vi "HEAVE UDP TRIAL.vi"() -> ()   [LabVIEW 2025]
panel:
  out "connection ID out":refnum<k16>
  in  "Checkbox":bool
  in  "Fine Tune Zone":dbl=10.0
  out "Pulse delta":dbl
  in  "seconds to wait 3":dbl=1.0 format="%#_6p"
  in  "Max_pos_limit":dbl=50000000.0
  in  "Min_pos_limit":dbl
  in  "i_limit":dbl=10.0
  in  "Max Step Linit":dbl=10.0
  in  "Init Step":dbl=10.0
  in  "pct_scale":dbl=100.0
  in  "Deadband":dbl=0.1
  in  "Kd":dbl
  in  "Ki":dbl
  in  "Kp":dbl=1.0
  out "Current Position":dbl
  in  "Set Load":dbl
  in  "Current Load":dbl
  out "Node Id":u8
  in  "PID SPEED":sgl=80000.0
  in  "PID":bool
  in  "seconds to wait 2":dbl=0.2 format="%#_6p"
  out "Pulse Output":dbl
  out "Trigger":dbl
  in  "Low Command":dbl
  in  "High Command":dbl=10000.0
  in  "Time Low":dbl=1.5
  in  "Time High":dbl=1.5
  in  "dt":dbl=0.01
  out "fwMinor":u8
  out "fwMajor":u8
  out "faultCode":u16
  out "SURGE POSE":sgl format="%#.6f"
  out "HEAVE POSE":sgl format="%#.6f"
  out "Homed":u8
  out "State":u8
  out "Ack ID":u16
  in  "Write":bool
  in  "Read":bool
  in  "seconds to wait":dbl=0.001 format="%#_6p"
  in  "SPEED":sgl=10000.0
  in  "Distance":sgl=10000.0
  in  "Mode Command":u8=2
  out "Sequence ID":u16=7
  out "string 2":string
  in  "Stop Button":bool
  in  "Server Name":string="192.168.1.10"
  out "data out 2":string
  # "0100 0100 0000 0000 0000 0000 0000 00"
  # "0100 0100 0000 0000 0000 0000 0000 0000"
  # "0500 0501 40C2 0C48 0000 0000 0000 0100"
  # "0300 0301 00CB E547 0000 0000 0000 0100"
  # "Home"
  # "0100 0100 0000 0000 0000 00"
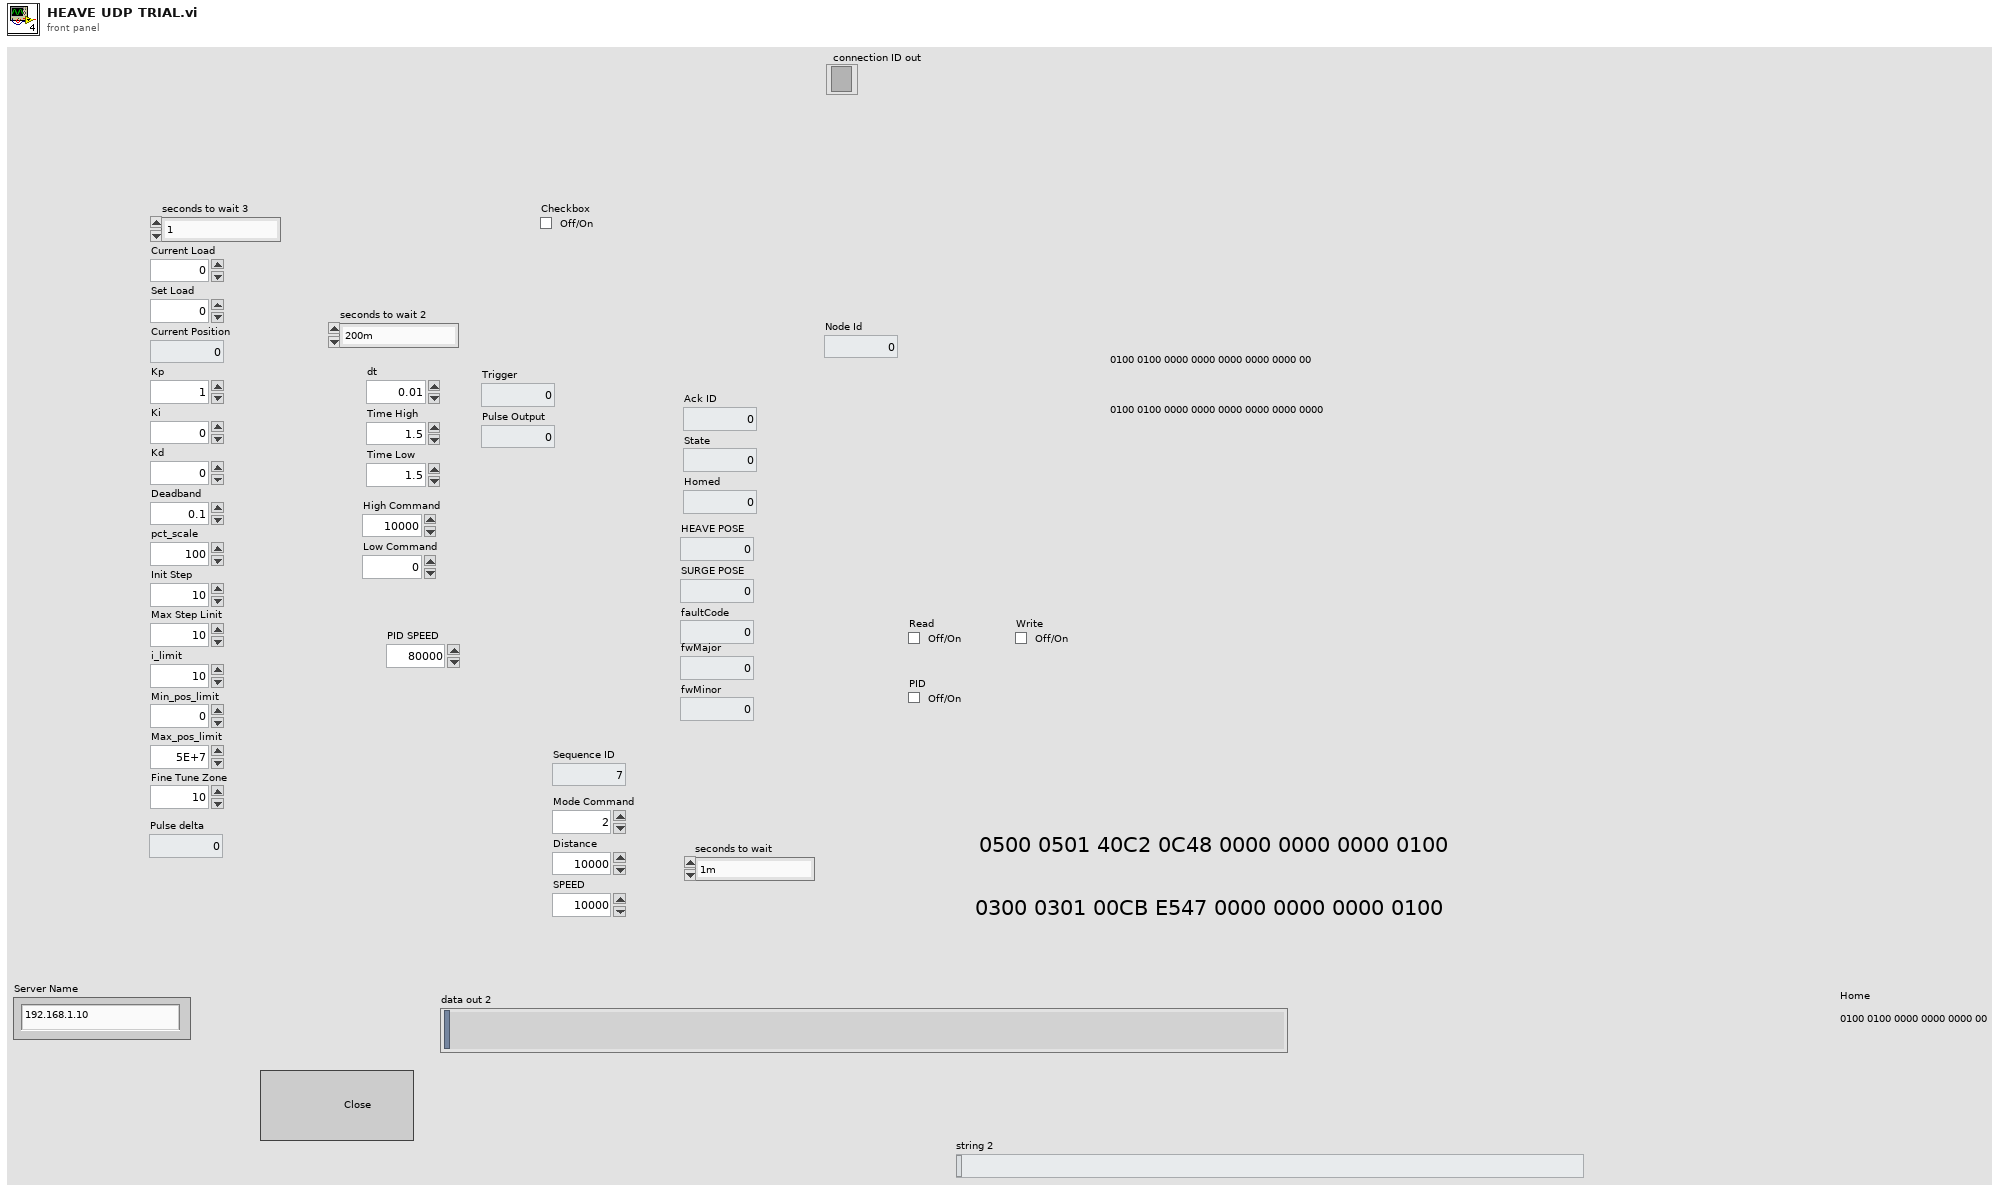
[diagram p1: front panel]
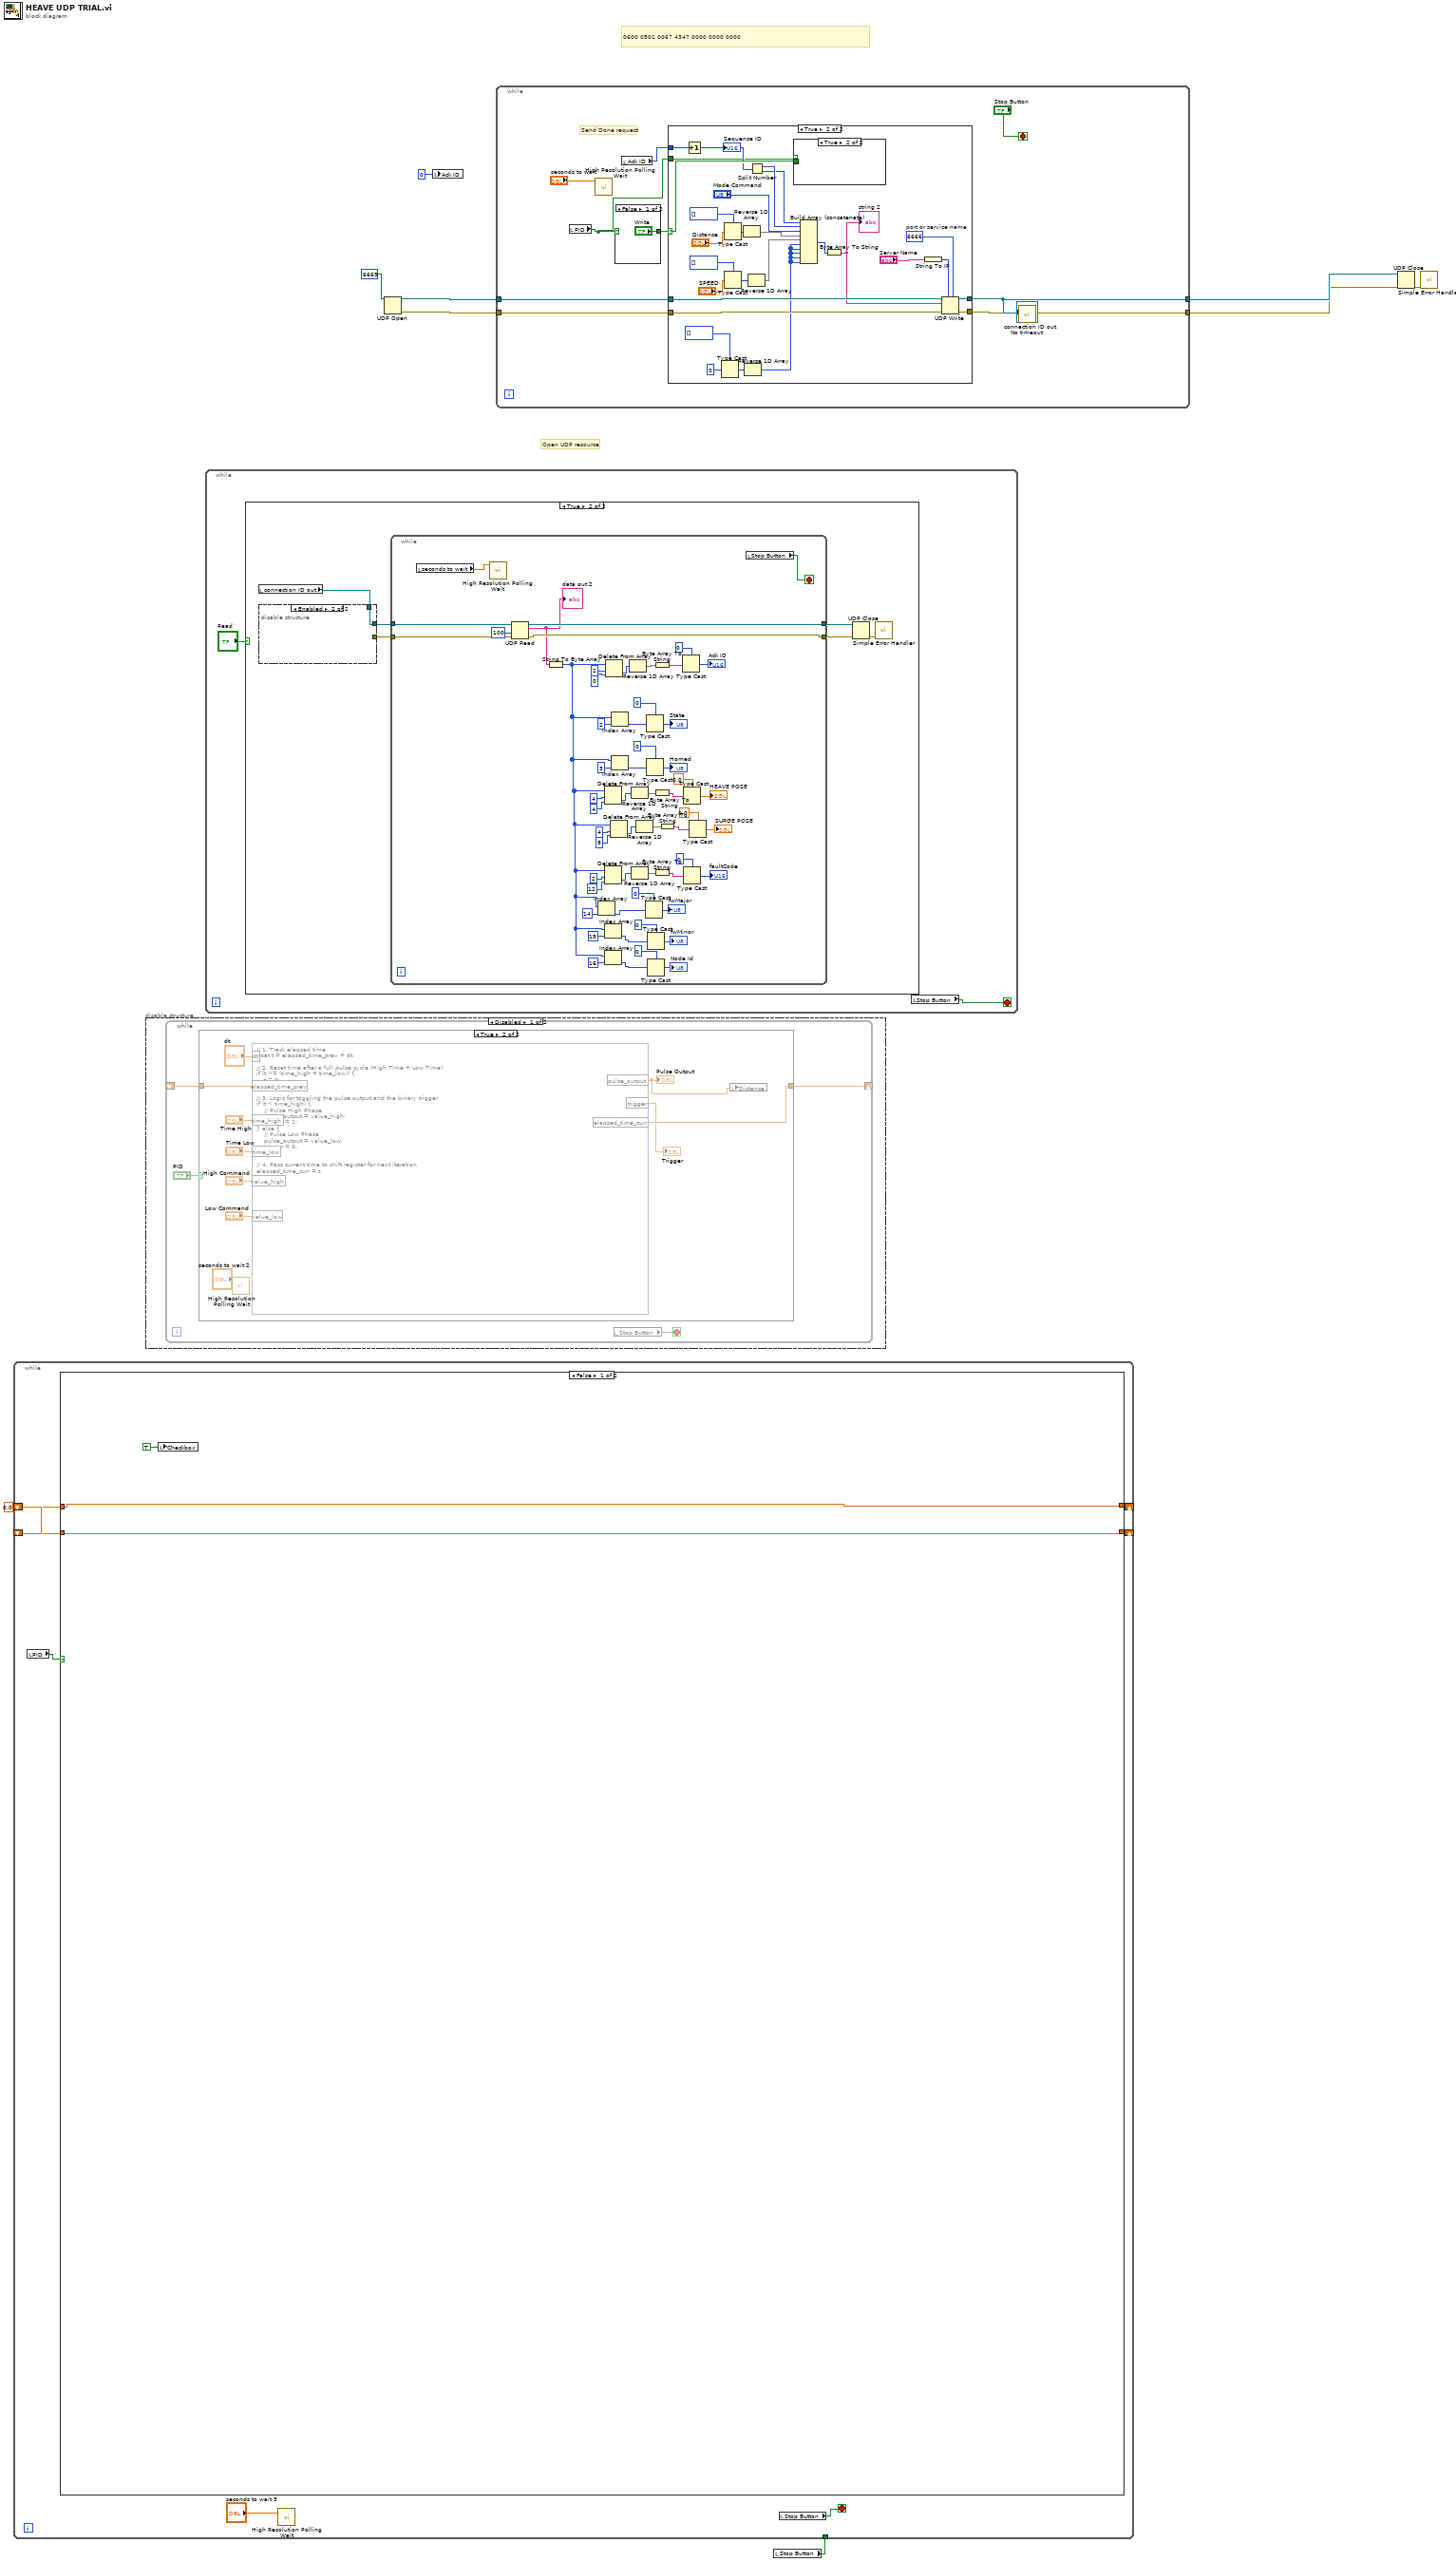
[diagram p0: block diagram]
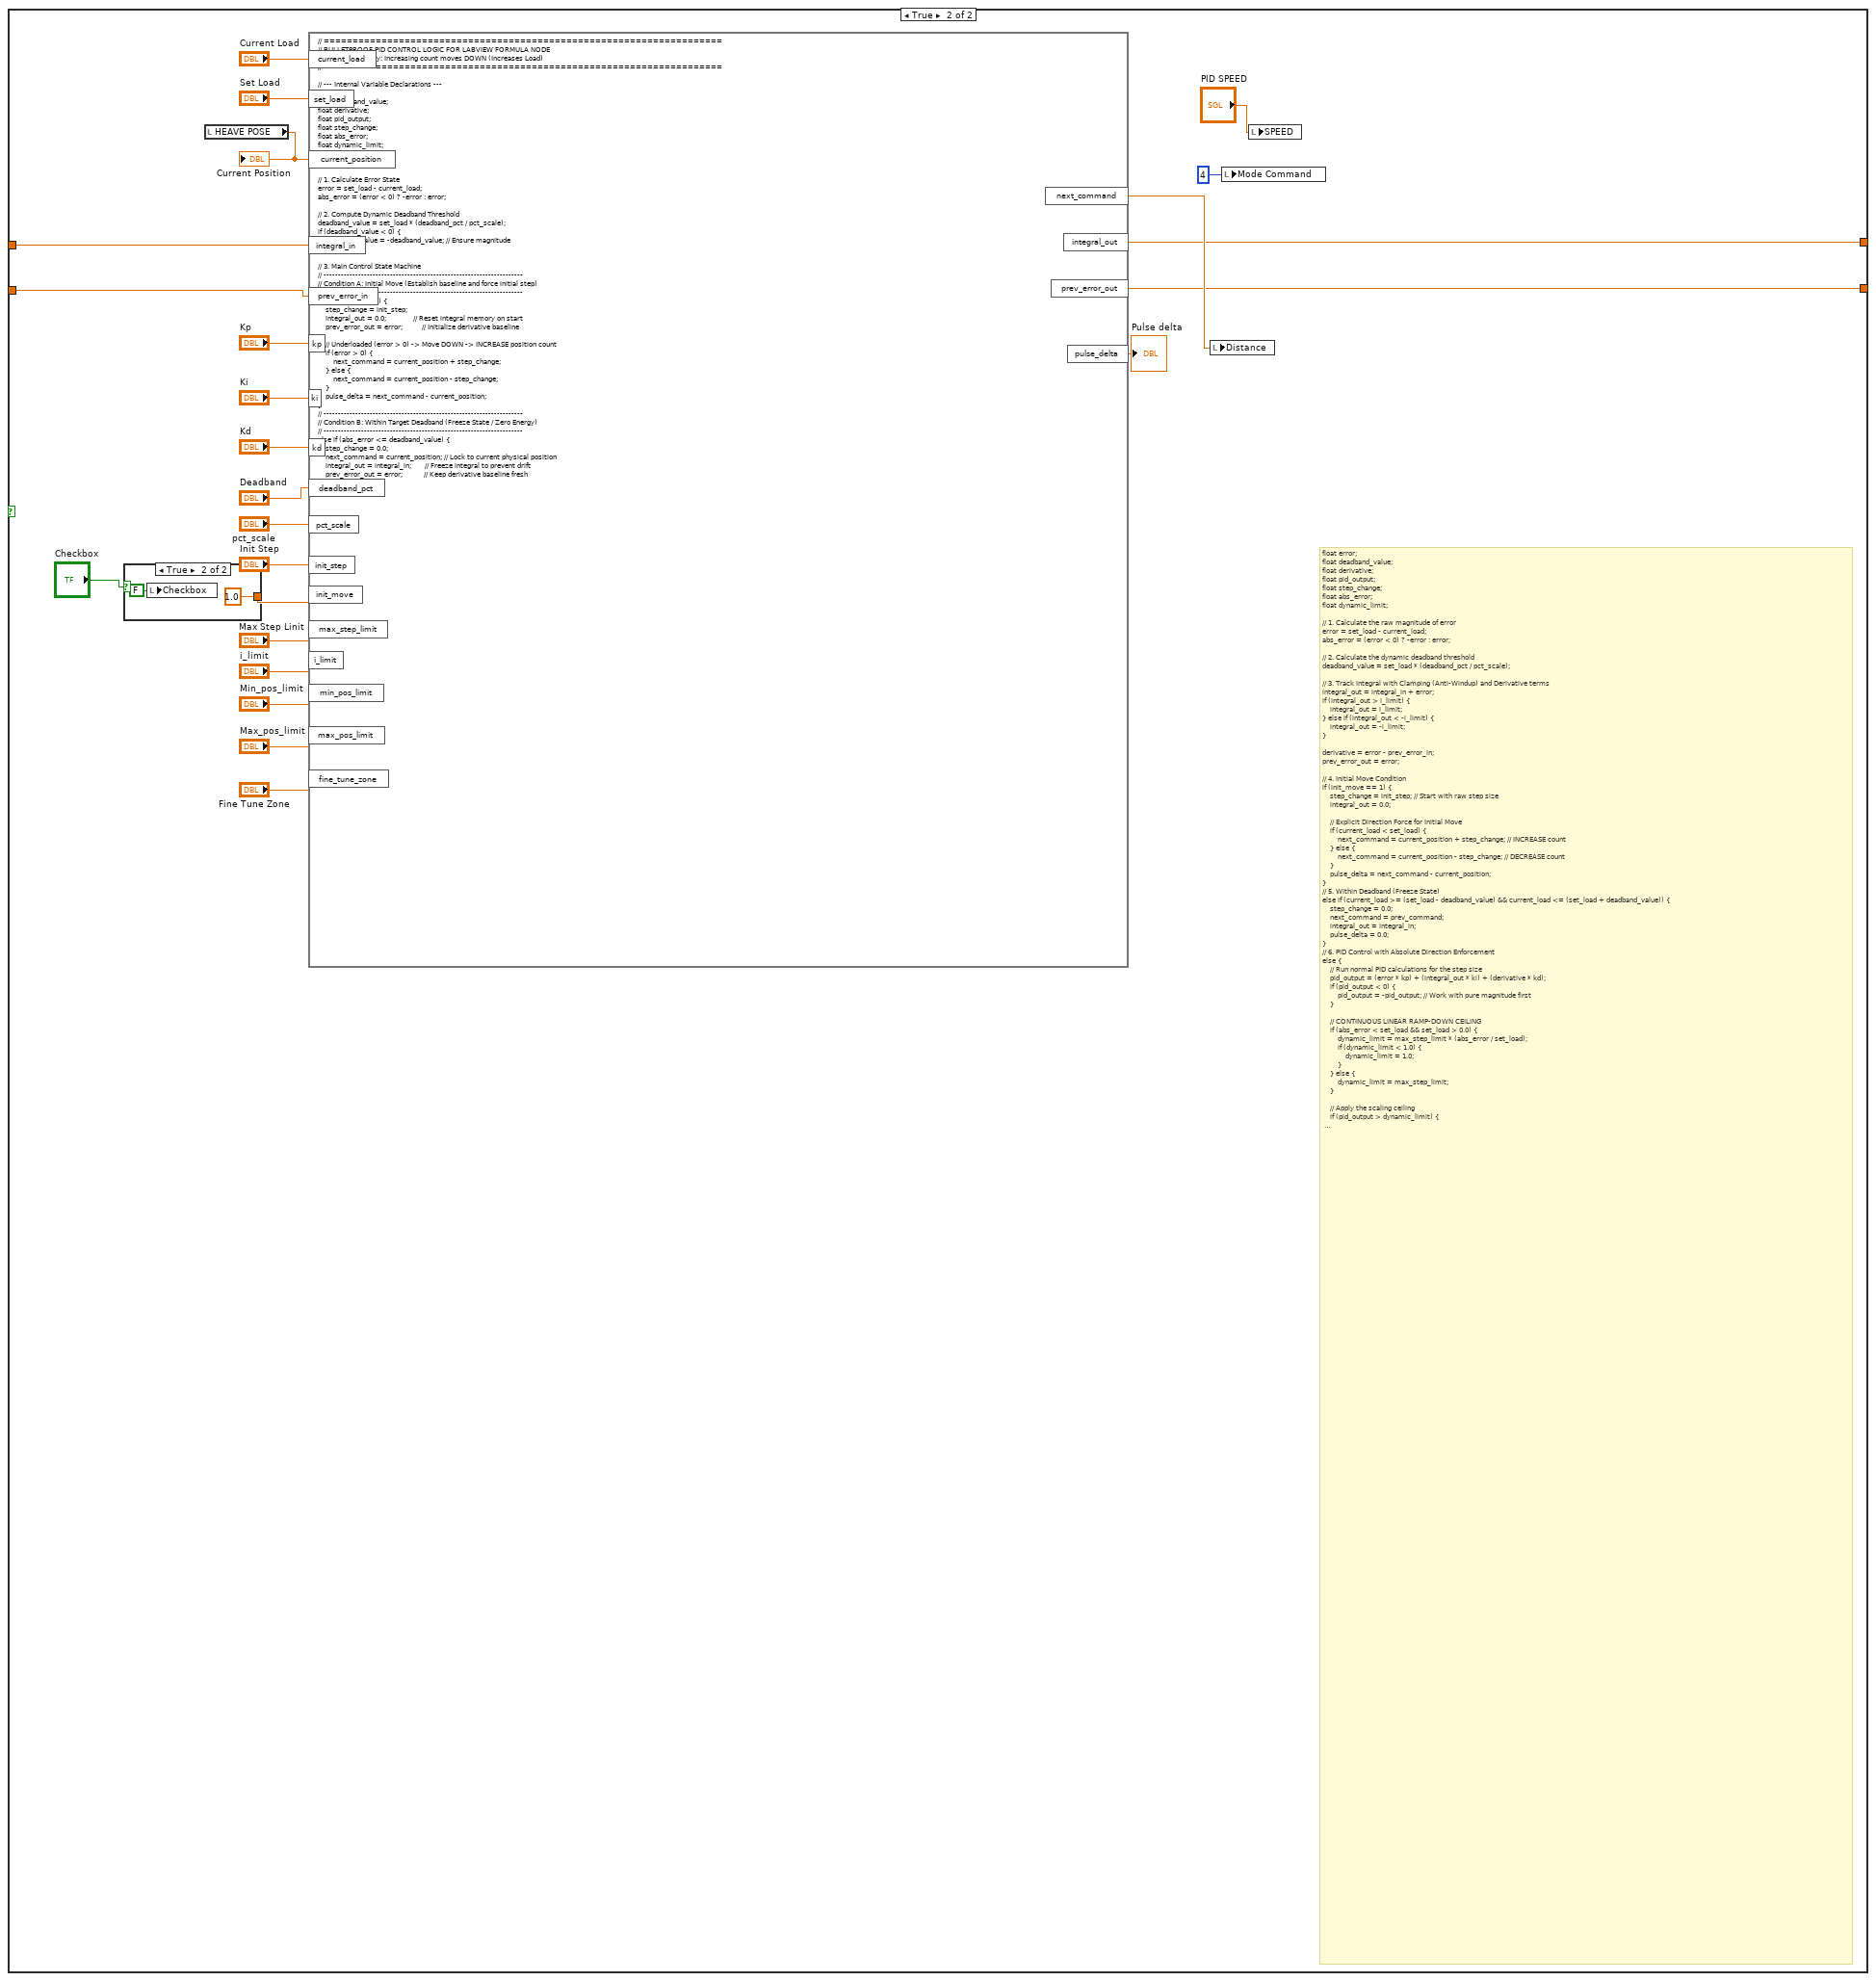
[diagram p2: hidden frame]
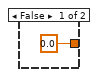
[diagram p3: hidden frame]
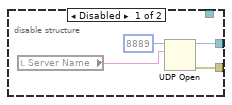
[diagram p7: hidden frame]
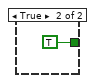
[diagram p8: hidden frame]
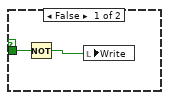
[diagram p10: hidden frame]
diagram:
  w1 = 0.0 ("integral_out")
  # "0600 0501 0067 4347 0000 0000 0000"
  # "Open UDP resource"
  n1 = disable-structure shown="Disabled" {
    frame Disabled {
      n2 = while {
        shift-right: [w11] -> _
        shift-left: _ -> [w12]
        stop <- w13 stop-if-true
        n3 = case shown="True" "PID" {
          tunnel: w12 -> [w14 w23]
          tunnel: [w14 w22] -> w11
          frame False {
          }
          frame True {
            n4 = call <vilib>:"High Resolution Polling Wait.vi"("seconds to wait"="seconds to wait 2") -> ()  [unwired: 10 in, 1 out]
            n5 = formula code="// 1. Track elapsed time\nfloat t = elapsed_time_prev + dt;\n\n// 2. Reset time after a full pulse cycle (High Time + Low Time)\nif (t >= (time_high + time_low)) {\n    t = 0;\n}\n\n// 3. Logic for toggling the pulse output and the binary trigger\nif (t < time_high) {\n    // Pulse High Phase\n    pulse_output = value_high;\n    trigger = 1; \n} else {\n    // Pulse Low Phase\n    pulse_output = value_low;\n    trigger = 0;\n}\n\n// 4. Pass current time to shift register for next iteration\nelapsed_time_curr = t;"("dt"="dt", "elapsed_time_prev"=w23, "time_high"="Time High", "time_low"="Time Low", "value_high"="High Command", "value_low"="Low Command") -> ("pulse_output"=w15:dbl, "trigger"=→"Trigger":dbl, "elapsed_time_curr"=w22:dbl)
            "Pulse Output" <- w15
            n6 = local write "Distance"(w15) -> ()
          }
        }
        n7 = local read "Stop Button"() -> (w13:bool)
      }
    }
    frame Enabled {
    }
  }
  n8 = while {
    stop <- w25 stop-if-true
    n9 = case shown="True" "Read" {
      frame False {
      }
      frame True {
        n10 = local read "connection ID out"() -> (w27:refnum<k16>)
        n11 = disable-structure shown="Enabled" {
          disable-tunnel: [w35 _] -> w32
          disable-tunnel: [w34 w37] -> w31
          disable-tunnel: w27 -> [_ w37]
          frame Disabled {
            n12 = local read "Server Name"() -> (w33:string)
            n13 = UDP Open(10:w33, 11:u16 8889 ("port")) -> (port=w34:refnum<k16>, 0:w35:errorcluster)  [unwired: 3 in, 1 out]
          }
          frame Enabled {
          }
        }
        n14 = while {
          tunnel: w32 -> [w94]
          tunnel: w31 -> [w93]
          tunnel: [w92] -> w29
          tunnel: [w90] -> w28
          stop <- w91 stop-if-true
          n15 = local read "seconds to wait"() -> (w88:dbl)
          n16 = call <vilib>:"High Resolution Polling Wait.vi"("seconds to wait"=w88) -> ()  [unwired: 10 in, 1 out]
          n17 = UDP Read(connection ID=w93, timeout ms (25000)=100, 8:w94) -> (data out=w47:string, error out=w92:errorcluster, 3:w90:refnum<k16>)  [unwired: 1 in, 2 out]
          "data out 2" <- w47
          n18 = String To Byte Array(string=w47) -> (unsigned byte array=w38:u8[])
          n19 = Index Array(array=w38, index=14) -> (element=w51:u8)
          n20 = Delete From Array(array=w38, length=4, index=4) -> (deleted portion=w43:u8[])  [unwired: 1 out]
          n21 = Delete From Array(array=w38, length=2, index=12) -> (deleted portion=w44:u8[])  [unwired: 1 out]
          n22 = Index Array(array=w38, index=15) -> (element=w48:u8)
          n23 = Index Array(array=w38, index=16) -> (element=w42:u8)
          n24 = Delete From Array(array=w38, length=2, index=0) -> (deleted portion=w45:u8[])  [unwired: 1 out]
          n25 = Delete From Array(array=w38, length=4, index=8) -> (deleted portion=w46:u8[])  [unwired: 1 out]
          n26 = Index Array(array=w38, index=2) -> (element=w79:u8)
          n27 = Index Array(array=w38, index=3) -> (element=w76:u8)
          n28 = Reverse 1D Array(array=w45) -> (reversed array=w85:u8[])
          n29 = Reverse 1D Array(array=w43) -> (reversed array=w71:u8[])
          n30 = Reverse 1D Array(array=w44) -> (reversed array=w58:u8[])
          n31 = Reverse 1D Array(array=w46) -> (reversed array=w66:u8[])
          n32 = Type Cast(type=u8 0, x=w51) -> (*(type *) &x=→"fwMajor":u8)
          n33 = Type Cast(type=u8 0, x=w79) -> (*(type *) &x=→"State":u8)
          n34 = Type Cast(type=u8 0, x=w76) -> (*(type *) &x=→"Homed":u8)
          n35 = Type Cast(type=u8 0, x=w48) -> (*(type *) &x=→"fwMinor":u8)
          n36 = Type Cast(type=u8 0, x=w42) -> (*(type *) &x=→"Node Id":u8)
          n37 = Byte Array To String(unsigned byte array=w71) -> (string=w69:string)
          n38 = Byte Array To String(unsigned byte array=w58) -> (string=w57:string)
          n39 = Byte Array To String(unsigned byte array=w85) -> (string=w83:string)
          n40 = Byte Array To String(unsigned byte array=w66) -> (string=w67:string)
          n41 = Type Cast(type=u16 0, x=w83) -> (*(type *) &x=→"Ack ID":u16)
          n42 = Type Cast(type=sgl 0.0, x=w69) -> (*(type *) &x=→"HEAVE POSE":sgl)
          n43 = Type Cast(type=u16 0, x=w57) -> (*(type *) &x=→"faultCode":u16)
          n44 = Type Cast(type=sgl 0.0, x=w67) -> (*(type *) &x=→"SURGE POSE":sgl)
          n45 = local read "Stop Button"() -> (w91:bool)
        }
        n46 = UDP Close(connection ID=w28, 8:w29) -> (error out=w30:errorcluster)  [unwired: 1 out]
        n47 = call <vilib>:"Simple Error Handler.vi"("error in (no error)"=w30) -> ()  [unwired: 4 in, 5 out]
      }
    }
    n48 = local read "Stop Button"() -> (w25:bool)
  }
  n49 = UDP Open(11:u16 6669 ("port")) -> (port=w9:refnum<k16>, 0:w8:errorcluster)  [unwired: 4 in, 1 out]
  n50 = local write "Ack ID"(u16 0 ("Ack ID")) -> ()
  n51 = while {
    tunnel: w9 -> [w104]
    tunnel: w8 -> [w103]
    tunnel: [w101] -> w6
    tunnel: [w102] -> w5
    stop <- "Stop Button" stop-if-true
    # "Send Done request"
    n52 = local read "PID"() -> (w95:bool)
    n53 = call <vilib>:"High Resolution Polling Wait.vi"("seconds to wait"="seconds to wait") -> ()  [unwired: 10 in, 1 out]
    n54 = case shown="False" w95 {
      tunnel: ["Write" TRUE ("Write")] -> w97
      frame False {
      }
      frame True {
      }
    }
    n55 = local read "Ack ID"() -> (w96:u16)
    n56 = case shown="True" w97 {
      selector: w97 -> [_ w116]
      tunnel: w104 -> [w107 w136]
      tunnel: w103 -> [w108 w135]
      tunnel: [w107 w132] -> w101
      tunnel: [w108 w131] -> w100
      tunnel: w96 -> [_ w115]
      tunnel: w95 -> [_ w113]
      frame False {
      }
      frame True {
        w130 = u16 6666  # port or service name
        n57 = Increment(x=w115) -> (x+1=w114:u16)
        "Sequence ID" <- w114
        n58 = Type Cast(type=u8[] [], x=u8 0) -> (*(type *) &x=w112:u8[])
        n59 = Type Cast(type=u8[] [], x="Distance") -> (*(type *) &x=w123:u8[])
        n60 = Type Cast(type=u8[] [], x="SPEED") -> (*(type *) &x=w124:u8[])
        n61 = Reverse 1D Array(array=w123) -> (reversed array=w128:u8[])
        n62 = Reverse 1D Array(array=w112) -> (reversed array=w109:u8[])
        n63 = Reverse 1D Array(array=w124) -> (reversed array=w129:u8[])
        n64 = Split Number(x=w114) -> (hi(x)=w127:u8, lo(x)=w126:u8)
        n65 = case shown="True" w113 {
          tunnel: w116 -> [w138 _]
          frame False {
            n66 = Not(x=w138) -> (.not. x?=w137:bool)
            n67 = local write "Write"(w137) -> ()
          }
          frame True {
          }
        }
        n68 = Build Array (concatenate)(w126, w127, "Mode Command", w128, w129, w109, w109, w109, w109, w109) -> (w125:u8[])
        n69 = Byte Array To String(unsigned byte array=w125) -> (string=w119:string)
        "string 2" <- w119
        n70 = String To IP(1:"Server Name") -> (0:w133:u32)
        n71 = UDP Write(address=w133, port or service name=w130, connection ID=w136, data in=w119, 8:w135) -> (error out=w131:errorcluster, 3:w132:refnum<k16>)  [unwired: 1 in]
      }
    }
    "connection ID out" <- w101
    n72 = call "No timeout.vi"("Error In"=w100) -> ("Error Out"=w102:errorcluster)  [unwired: 10 in]
  }
  n73 = local read "Stop Button"() -> (w2:bool)
  n74 = while {
    shift-right: [w144] -> _
    shift-left: w1 -> [w145]
    shift-right: [w142] -> _
    shift-left: w1 -> [w143]
    tunnel: w2 -> [_]
    stop <- w140 stop-if-true
    n75 = local read "PID"() -> (w139:bool)
    n76 = case shown="False" w139 {
      tunnel: w145 -> [w147 w171]
      tunnel: [w147 w170] -> w144
      tunnel: w143 -> [w148 w169]
      tunnel: [w148 w168] -> w142
      frame False {
        n77 = local write "Checkbox"(TRUE ("Checkbox")) -> ()
      }
      frame True {
        # "float error;\nfloat deadband_value;\nfloat derivative;\nfloat pid_output;\nfloat step_change;\nfloat abs_error;\nfloat dynamic_limit;\n\n// 1. Calculate the raw magnitude of error\nerror = set_load - current_load;\nabs_error = (error < 0) ? -error : error;\n\n// 2. Calculate the dynamic deadband threshold\ndeadband_value = set_load * (deadband_pct / pct_scale);\n\n// 3. Track Integral with Clamping (Anti-Windup) and Derivative terms\nintegral_out = integral_in + error;\nif (integral_out > i_limit) {\n    integral_out = i_limit;\n} else if (integral_out < -i_limit) {\n    integral_out = -i_limit;\n}\n\nderivative = error - prev_error_in;\nprev_error_out = error;\n\n// 4. Initial Move Condition\nif (init_move == 1) {\n    step_change = init_step; // Start with raw step size\n    integral_out = 0.0;\n    \n    // Explicit Direction Force for Initial Move\n    if (current_load < set_load) {\n        next_command = current_position + step_change; // INCREASE count\n    } else {\n        next_command = current_position - step_change; // DECREASE count\n    }\n    pulse_delta = next_command - current_position;\n}\n// 5. Within Deadband (Freeze State)\nelse if (current_load >= (set_load - deadband_value) && current_load <= (set_load + deadband_value)) {\n    step_change = 0.0;\n    next_command = prev_command;\n    integral_out = integral_in;\n    pulse_delta = 0.0;\n} \n// 6. PID Control with Absolute Direction Enforcement\nelse {\n    // Run normal PID calculations for the step size\n    pid_output = (error * kp) + (integral_out * ki) + (derivative * kd);\n    if (pid_output < 0) {\n        pid_output = -pid_output; // Work with pure magnitude first\n    }\n    \n    // CONTINUOUS LINEAR RAMP-DOWN CEILING\n    if (abs_error < set_load && set_load > 0.0) {\n        dynamic_limit = max_step_limit * (abs_error / set_load);\n        if (dynamic_limit < 1.0) {\n            dynamic_limit = 1.0;\n        }\n    } else {\n        dynamic_limit = max_step_limit;\n    }\n\n    // Apply the scaling ceiling\n    if (pid_output > dynamic_limit) {\n        step_change = dynamic_limit;\n    } else {\n        step_change = pid_output;\n    }\n    \n    // FORCED 1-COUNT PRECISION STEPPING BELOW THE THRESHOLD\n    if (abs_error <= fine_tune_zone) {\n        step_change = 1.0;\n    }\n\n    // -----------------------------------------------------------------\n    // CRITICAL FIX: ABSOLUTE DIRECTIONAL GUARANTEE\n    // -----------------------------------------------------------------\n    if (current_load < set_load) {\n        // Condition: Underloaded -> Motor count MUST increase\n        next_command = prev_command + step_change; \n    } else {\n        // Condition: Overloaded -> Motor count MUST decrease\n        next_command = prev_command - step_change; \n    }\n    \n    pulse_delta = next_command - prev_command;\n}\n\n// 7. Hard Absolute Safety Boundary Guard\nif (next_command > max_pos_limit) {\n    next_command = max_pos_limit;\n    pulse_delta = next_command - prev_command;\n} else if (next_command < min_pos_limit) {\n    next_command = min_pos_limit;\n    pulse_delta = next_command - prev_command;\n}"
        n78 = case shown="True" "Checkbox" {
          tunnel: [0.0 ("Init Move") 1.0 ("Init Move")] -> w159
          frame False {
          }
          frame True {
            n79 = local write "Checkbox"(FALSE ("Checkbox")) -> ()
          }
        }
        n80 = local read "HEAVE POSE"() -> (w154:sgl)
        "Current Position" <- w154
        n81 = formula code="// =====================================================================\n// BULLETPROOF PID CONTROL LOGIC FOR LABVIEW FORMULA NODE\n// Direction Polarity: Increasing count moves DOWN (Increases Load)\n// =====================================================================\n\n// --- Internal Variable Declarations ---\nfloat error;\nfloat deadband_value;\nfloat derivative;\nfloat pid_output;\nfloat step_change;\nfloat abs_error;\nfloat dynamic_limit;\nfloat pid_sign;\nfloat abs_pid;\n\n// 1. Calculate Error State\nerror = set_load - current_load;\nabs_error = (error < 0) ? -error : error;\n\n// 2. Compute Dynamic Deadband Threshold\ndeadband_value = set_load * (deadband_pct / pct_scale);\nif (deadband_value < 0) {\n    deadband_value = -deadband_value; // Ensure magnitude\n}\n\n// 3. Main Control State Machine\n// ---------------------------------------------------------------------\n// Condition A: Initial Move (Establish baseline and force initial step)\n// ---------------------------------------------------------------------\nif (init_move == 1) {\n    step_change = init_step; \n    integral_out = 0.0;              // Reset integral memory on start\n    prev_error_out = error;          // Initialize derivative baseline\n    \n    // Underloaded (error > 0) -> Move DOWN -> INCREASE position count\n    if (error > 0) {\n        next_command = current_position + step_change;\n    } else {\n        next_command = current_position - step_change;\n    }\n    pulse_delta = next_command - current_position;\n}\n// ---------------------------------------------------------------------\n// Condition B: Within Target Deadband (Freeze State / Zero Energy)\n// ---------------------------------------------------------------------\nelse if (abs_error <= deadband_value) {\n    step_change = 0.0;\n    next_command = current_position; // Lock to current physical position\n    integral_out = integral_in;       // Freeze integral to prevent drift\n    prev_error_out = error;           // Keep derivative baseline fresh\n    pulse_delta = 0.0;\n} \n// ---------------------------------------------------------------------\n// Condition C: Active PID Control Zone\n// ---------------------------------------------------------------------\nelse {\n    // A. Track Integral with strict Anti-Windup Limits\n    integral_out = integral_in + error;\n    if (integral_out > i_limit) {\n        integral_out = i_limit;\n    } else if (integral_out < -i_limit) {\n        integral_out = -i_limit;\n    }\n\n    // B. Calculate Derivative (Tracks rate of change of error)\n    derivative = error - prev_error_in;\n    prev_error_out = error; // Pass to next iteration\n\n    // C. Execute Raw PID Equation\n    pid_output = (error * kp) + (integral_out * ki) + (derivative * kd);\n    \n    // D. Extract Mathematical Sign and Magnitude\n    pid_sign = (pid_output >= 0) ? 1.0 : -1.0;\n    abs_pid = (pid_output < 0) ? -pid_output : pid_output;\n\n    // E. Continuous Linear Ramp-Down Ceiling\n    if (abs_error < set_load && set_load > 0.0) {\n        dynamic_limit = max_step_limit * (abs_error / set_load);\n        if (dynamic_limit < 1.0) {\n            dynamic_limit = 1.0; // Ensure at least a minimum microstep ceiling\n        }\n    } else {\n        dynamic_limit = max_step_limit;\n    }\n\n    // F. Apply Dynamic Ceiling to PID output magnitude\n    if (abs_pid > dynamic_limit) {\n        step_change = dynamic_limit;\n    } else {\n        step_change = abs_pid;\n    }\n    \n    // G. Forced 1-Count Precision Stepping in Fine-Tune Zone\n    if (abs_error <= fine_tune_zone) {\n        step_change = 1.0;\n    }\n\n    // H. Apply Step Vector directly relative to physical position\n    // Positive Error -> Positive Sign -> Increases count (Moves Downward to Load)\n    // Negative Derivative (Braking) -> Flips Sign -> Decreases count (Brakes Velocity)\n    next_command = current_position + (step_change * pid_sign);\n    pulse_delta = next_command - current_position;\n}\n\n// 4. Hard Structural Boundaries & Safety Guards\n// ---------------------------------------------------------------------\nif (next_command > max_pos_limit) {\n    next_command = max_pos_limit;\n    pulse_delta = next_command - current_position;\n} else if (next_command < min_pos_limit) {\n    next_command = min_pos_limit;\n    pulse_delta = next_command - current_position;\n}"("current_load"="Current Load", "set_load"="Set Load", "current_position"=w154, "integral_in"=w171, "prev_error_in"=w169, "kp"="Kp", "ki"="Ki", "kd"="Kd", "deadband_pct"="Deadband", "pct_scale"="pct_scale", "init_step"="Init Step", "init_move"=w159, "max_step_limit"="Max Step Linit", "i_limit"="i_limit", "min_pos_limit"="Min_pos_limit", "max_pos_limit"="Max_pos_limit", "fine_tune_zone"="Fine Tune Zone") -> ("next_command"=w172:dbl, "integral_out"=w170:dbl, "prev_error_out"=w168:dbl, "pulse_delta"=→"Pulse delta":dbl)
        n82 = local write "Distance"(w172) -> ()
        n83 = local write "Mode Command"(u8 4 ("Mode Command")) -> ()
        n84 = local write "SPEED"("PID SPEED") -> ()
      }
    }
    n85 = call <vilib>:"High Resolution Polling Wait.vi"("seconds to wait"="seconds to wait 3") -> ()  [unwired: 10 in, 1 out]
    n86 = local read "Stop Button"() -> (w140:bool)
  }
  n87 = UDP Close(connection ID=w6, 8:w5) -> (error out=w4:errorcluster)  [unwired: 1 out]
  n88 = call <vilib>:"Simple Error Handler.vi"("error in (no error)"=w4) -> ()  [unwired: 4 in, 5 out]
